vi "STAGE+mono+counter_edit1.vi"() -> ()   [LabVIEW 2017]
panel:
  in  "Integrating time, 10^-7 sec":dbl=10000000.0
  out "Timeout 2":bool
  in  "scan from":i32=2600
  in  "scan to":i32=4000
  in  "?":bool
  in  "Exit Labview":bool
  in  "step size":dbl=10.0 min=0.0
  in  "Name of measurement (optional)":string
  in  "?":bool
  out "Spectrum":waveform(dbl)(graph)
  out "Counts":i32
  in  "Background scan":bool=TRUE
  in  "value (0)":dbl=-9.0
  in  "number of disc steps":i32=1
  in  "Background scan 2":bool=TRUE
  out "Current WL Wavelength  2":u16 caption="Current Wavelength"
  out "Grt# 2":u8=1 min=1 max=3 step=1
  out "Blaze (nm)":u32=300
  out "Groove/mm":u32=1200
  in  "?":bool
  in  "Channel B Input":u16(ring)=2 items=["Input 1"=1, "Input 2"=2]
  in  "Trigger mode":u16(ring) items=["10 MHz"=0, "Input 2"=2, "Input T"=3]
  out "Current WL Wavelength":u16 caption="Current Wavelength"
  in  "Integrating time, 10^-7 sec":dbl=10000000.0
  in  "gate A mode (CW:0)":i16(slide) scale=0.0..2.0 scale format="%.2f"
  in  "Channel A Input":u16(ring)=1 items=["10 MHz", "Input 1"]
  in  "Time between measurements\n at one point (s)/Dwell Time":dbl=0.002 min=0.002 max=60.0 step=0.001
  in  "Number of Measurements\n to take at one point/ Number of Periods":u16=1 min=1 max=2000 step=1
  in  "Count Mode":u16(ring) items=["A,B for Preset T", "A-B for Preset T", "A+B for Preset T", "A for Preset B"]
  in  "GPIB address":string="23"
  out "Timeout":bool
  out "Serial":u32=12345
  out "Grt#":u8=1 min=1 max=3 step=1
  out "Blaze (nm)":u32=300
  out "Groove/mm":u32=1200
  out "time delay":u32=450000 min=1
  out "Mono port":T1(ring)
  in  "Get position":bool
  out "Position status":dbl format="%.3f"
  in  "Target position":dbl format="%.3f"
  in  "Move":bool
  in  "Motor OFF":bool
  in  "Motor ON":bool
  in  "Step Size [um]":i32=10
  in  "Axis":i32=1
  in  "Rep Rate [Hz]":dbl=500.0
  out "Shots":dbl
  in  "Averaging Time [s]":dbl=0.1
  out "Current Point":i32
  out "Slide":i32(slide) scale=0.0..100.0
  out "Current Position [mm]":dbl
  in  "Axis initial position [mm]":dbl
  out "Axis final Position [mm]":dbl
  in  "Data Points (100 default)":i32=100
  in  "Collect Data!":bool
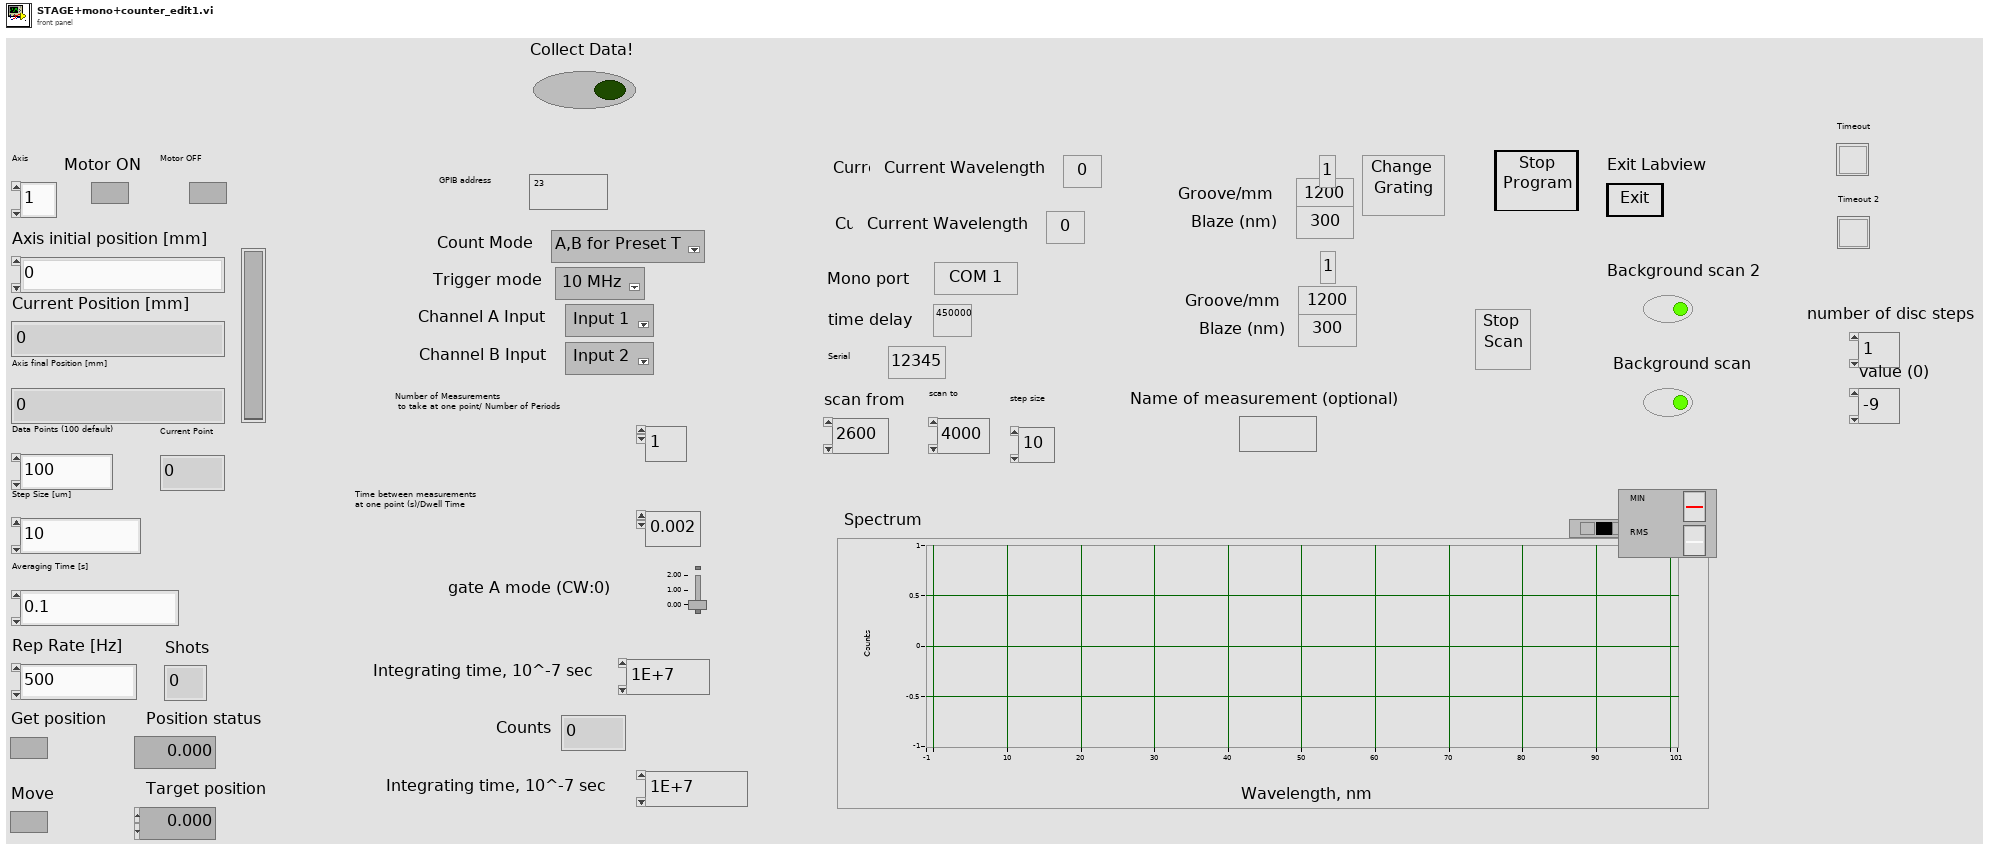
[diagram p1: front panel]
types:
  T1 = enum8{"COM 1", "COM 2", "COM 3", "COM 4", "COM 5", "COM 6", "COM 7", "COM 8", "COM 9"}
  T2 = cluster{"input XON/XOFF":bool, "input HW Handshake":bool, "input alt HW HShk":bool, "output XON/XOFF":bool, "output HW Handshake":bool, "output alt HW HShk":bool, "XOFF byte":u8, "XON byte":u8, "parity error byte":u16}
  T3 = enum16{"no parity", "odd parity", "even parity", "mark parity", "space parity"}
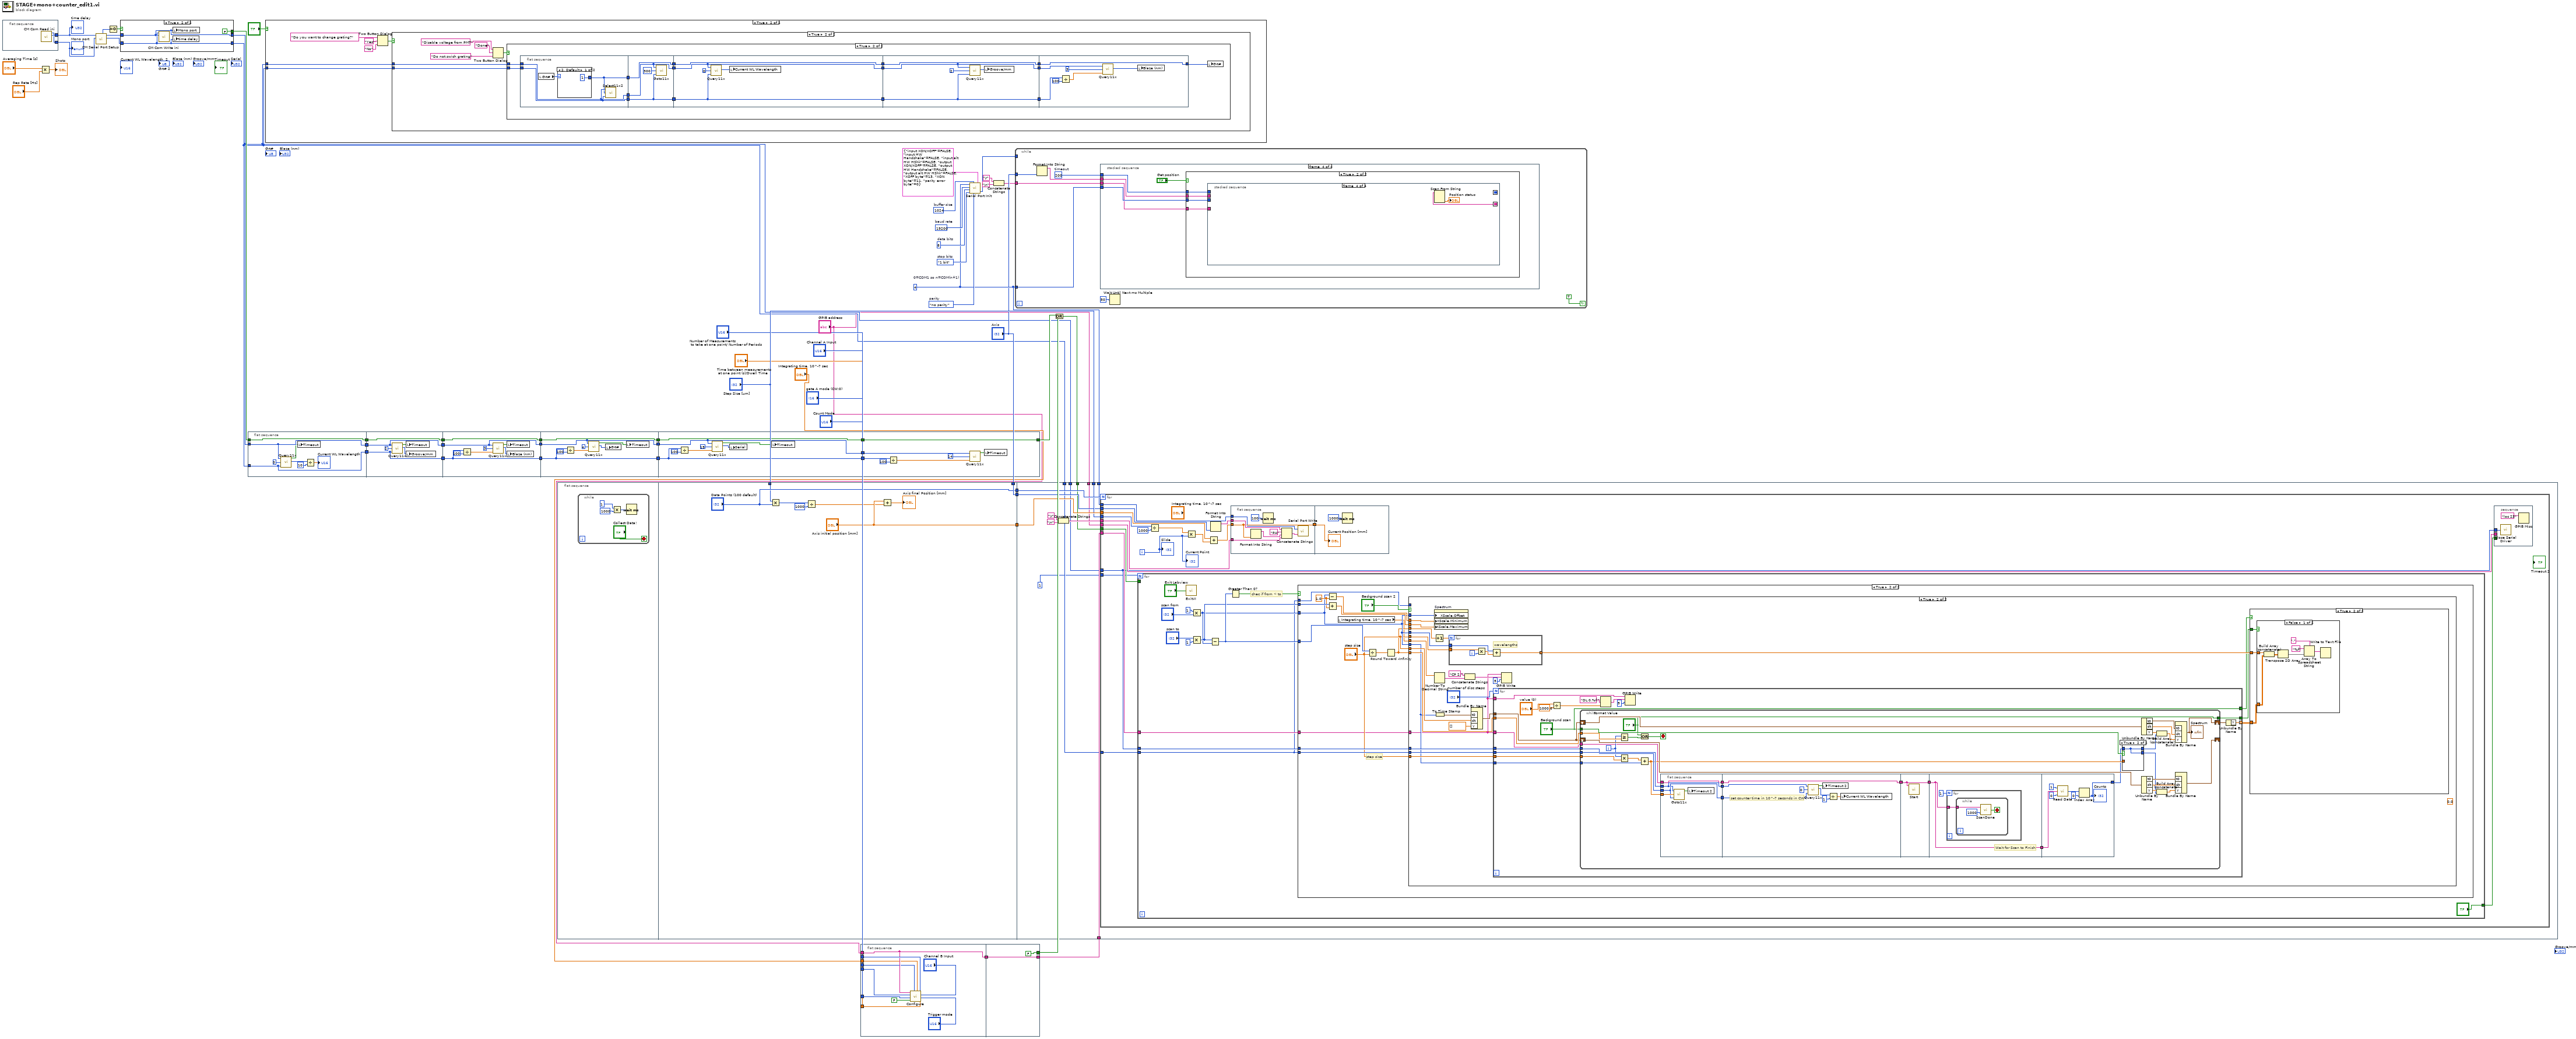
[diagram p0: block diagram]
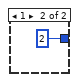
[diagram p5: hidden frame]
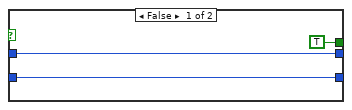
[diagram p6: hidden frame]
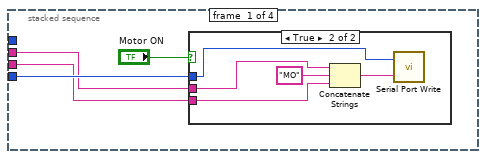
[diagram p7: hidden frame]
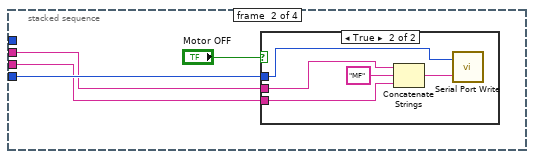
[diagram p9: hidden frame]
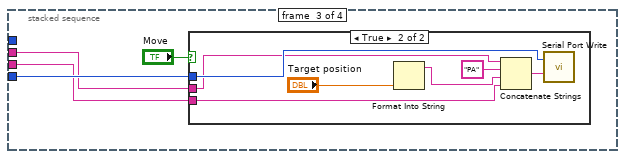
[diagram p11: hidden frame]
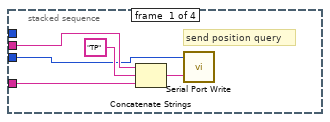
[diagram p14: hidden frame]
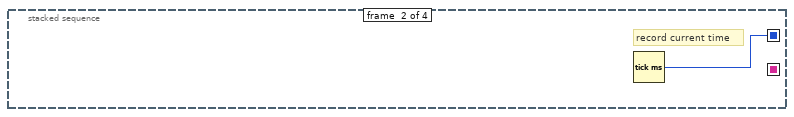
[diagram p15: hidden frame]
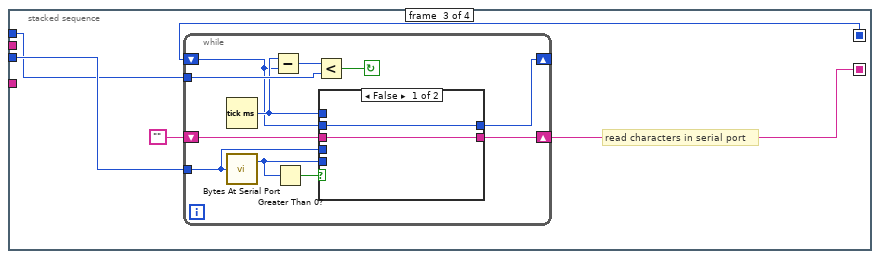
[diagram p16: hidden frame]
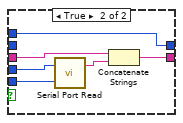
[diagram p17: hidden frame]
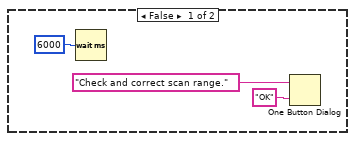
[diagram p18: hidden frame]
diagram:
  w46 = u32 19200  # baud rate
  w45 = u16 8  # data bits
  w44 = enum16{"1 bit", "1.5 bits", "2 bits"}."1 bit"  # stop bits
  w49 = T3."no parity"  # parity
  w43 = 4  # 0=COM1 so n=COM(n+1)
  w48 = u16 1024  # buffer size
  n1 = flat-sequence {
    tunnel: [w58] -> w21
    tunnel: [w57] -> w20
    frame #0 {
      n2 = call "CM Com Read ini.vi"() -> ("Mono port"=w57:T1, "time delay1"=w58:u32)  [unwired: 7 in]
    }
  }
  n3 = Multiply(x="Averaging Time [s]", y="Rep Rate [Hz]") -> (x*y=→"Shots":dbl)
  n4 = call "CM Serial Port Setup.vi"("COM port"=w20, "time delay"=w21) -> ("time delay1"=w16:u32, "DK port Out"=w17:T1, "error code"=w19:i32)  [unwired: 7 in]
  n5 = Equal To 0?(x=w19) -> (x = 0?=w18:bool)
  n6 = case shown="True" w18 {
    tunnel: w17 -> [w61 w64]
    tunnel: w16 -> [w60 w63]
    tunnel: [w61 w64] -> w3
    tunnel: [w60 w63] -> w2
    tunnel: [TRUE FALSE] -> w15
    frame False {
    }
    frame True {
      n7 = call "CM Com Write ini.vi"("time delay1"=w64, "Mono port"=w63) -> ()  [unwired: 7 in]
      n8 = local write "Mono port"(w64) -> ()
      n9 = local write "time delay"(w63) -> ()
    }
  }
  n10 = flat-sequence {
    tunnel: w2 -> [w70]
    tunnel: [w70] -> w37
    tunnel: w3 -> [w72]
    tunnel: [w72] -> w36
    tunnel: w15 -> [w68]
    tunnel: [w68] -> w35
    tunnel: w37 -> [w75]
    tunnel: [w75] -> w34
    tunnel: w36 -> [w77]
    tunnel: [w77] -> w33
    tunnel: w35 -> [w73]
    tunnel: [w73] -> w32
    tunnel: w34 -> [w85]
    tunnel: [w85] -> w31
    tunnel: w33 -> [w82]
    tunnel: [w82] -> w30
    tunnel: w32 -> [w79]
    tunnel: [w79] -> w29
    tunnel: w31 -> [w93]
    tunnel: [w93] -> w28
    tunnel: w30 -> [w90]
    tunnel: [w90] -> w27
    tunnel: w29 -> [w87]
    tunnel: [w87] -> w26
    tunnel: w28 -> [w101]
    tunnel: [w101] -> w25
    tunnel: w27 -> [w98]
    tunnel: [w98] -> w24
    tunnel: w26 -> [w95]
    tunnel: [w95] -> w23
    tunnel: w25 -> [w108]
    tunnel: w24 -> [w105]
    tunnel: [w103] -> w9
    tunnel: w23 -> [w103]
    frame #0 {
      n11 = call "Query11x.vi"("port number"=w72, "QUERY"=u16 0, "time delay"=w70) -> ("timeout"=w69:bool, "STATUS MESSAGE"=w67:u16)  [unwired: 2 out]
      n12 = local write "Timeout"(w69) -> ()
      n13 = Divide(x=w67, y=10 ("Numeric")) -> (x/y=→"Current WL Wavelength":dbl)
    }
    frame #1 {
      n14 = call "Query11x.vi"("port number"=w77, "QUERY"=u16 2, "time delay"=w75) -> ("timeout"=w74:bool, "STATUS MESSAGE"=w76:u16)  [unwired: 2 out]
      n15 = local write "Timeout"(w74) -> ()
      n16 = local write "Groove/mm"(w76) -> ()
    }
    frame #2 {
      n17 = Divide(x=w85, y=i16 100 ("device (1)")) -> (x/y=w83:dbl)
      n18 = call "Query11x.vi"("port number"=w82, "QUERY"=u16 3, "time delay"=w83) -> ("timeout"=w80:bool, "STATUS MESSAGE"=w81:u16)  [unwired: 2 out]
      n19 = local write "Timeout"(w80) -> ()
      n20 = local write "Blaze (nm)"(w81) -> ()
    }
    frame #3 {
      n21 = Divide(x=w93, y=i16 100 ("device (1)")) -> (x/y=w91:dbl)
      n22 = call "Query11x.vi"("port number"=w90, "QUERY"=u16 4, "time delay"=w91) -> ("timeout"=w88:bool, "STATUS MESSAGE"=w89:u16)  [unwired: 2 out]
      n23 = local write "Grt#"(w89) -> ()
      n24 = local write "Timeout"(w88) -> ()
    }
    frame #4 {
      n25 = Divide(x=w101, y=i16 100 ("device (1)")) -> (x/y=w99:dbl)
      n26 = call "Query11x.vi"("port number"=w98, "QUERY"=u16 19, "time delay"=w99) -> ("timeout"=w96:bool, "STATUS MESSAGE"=w97:u16)  [unwired: 2 out]
      n27 = local write "Serial"(w97) -> ()
      n28 = local write "Timeout"(w96) -> ()
    }
    frame #5 {
      n29 = Divide(x=w108, y=i16 100 ("device (1)")) -> (x/y=w106:dbl)
      n30 = call "Query11x.vi"("port number"=w105, "QUERY"=u16 14, "time delay"=w106) -> ("timeout"=w104:bool)  [unwired: 3 out]
      n31 = local write "Timeout"(w104) -> ()
    }
  }
  n32 = case shown="True" "?" {
    tunnel: w2 -> [_ w111]
    tunnel: w3 -> [_ w110]
    frame False {
    }
    frame True {
      n33 = Two Button Dialog(message="Do you want to change grating?", 1:"No" ("F button name (\"Cancel\")"), 2:"Yes" ("T button name (\"OK\")")) -> (T button?=w112:bool)
      n34 = case shown="True" w112 {
        tunnel: w111 -> [_ w117]
        tunnel: w110 -> [_ w116]
        frame False {
        }
        frame True {
          n35 = Two Button Dialog(message="Disable voltage from PMT", 1:"Do not swich grating" ("F button name (\"Cancel\")"), 2:"Done" ("T button name (\"OK\")")) -> (T button?=w118:bool)
          n36 = case shown="True" w118 {
            tunnel: w117 -> [_ w136]
            tunnel: w116 -> [_ w135]
            frame False {
            }
            frame True {
              n37 = flat-sequence {
                tunnel: w136 -> [w140]
                tunnel: [w140] -> w133
                tunnel: w135 -> [w139]
                tunnel: [w139] -> w132
                tunnel: [w137] -> w131
                tunnel: w133 -> [w144]
                tunnel: [w144] -> w130
                tunnel: w132 -> [w145]
                tunnel: [w145] -> w129
                tunnel: w131 -> [w143]
                tunnel: [w143] -> w128
                tunnel: w130 -> [w151]
                tunnel: [w151] -> w127
                tunnel: w129 -> [w150]
                tunnel: [w150] -> w126
                tunnel: w128 -> [w147]
                tunnel: [w147] -> w125
                tunnel: w127 -> [w154]
                tunnel: [w154] -> w124
                tunnel: w126 -> [w155]
                tunnel: [w155] -> w123
                tunnel: w125 -> [w152]
                tunnel: [w152] -> w122
                tunnel: w124 -> [w159]
                tunnel: w123 -> [w160]
                tunnel: [w157] -> w134
                tunnel: w122 -> [w157]
                frame #0 {
                  n38 = local read "Grt#"() -> (w138:u8)
                  n39 = case shown="2, Default" w138 {
                    tunnel: [1 2] -> w137
                    frame 2, Default {
                    }
                    frame 1 {
                    }
                  }
                  n40 = call "Select11x2.vi"("time delay"=w140, "NEW GRT?"=w137, "port number"=w139) -> ()  [unwired: 3 out]
                }
                frame #1 {
                  n41 = call "Goto11x.vi"("time delay"=w144, "WAVELENGTH"=u16 300, "port number"=w145) -> ()  [unwired: 3 out]
                }
                frame #2 {
                  n42 = call "Query11x.vi"("port number"=w150, "QUERY"=u16 0, "time delay"=w151) -> ("STATUS MESSAGE"=w148:u16)  [unwired: 3 out]
                  n43 = local write "Current WL Wavelength"(w148) -> ()
                }
                frame #3 {
                  n44 = call "Query11x.vi"("port number"=w155, "QUERY"=u16 2, "time delay"=w154) -> ("STATUS MESSAGE"=w153:u16)  [unwired: 3 out]
                  n45 = local write "Groove/mm"(w153) -> ()
                }
                frame #4 {
                  n46 = Divide(x=w159, y=i16 100 ("device (1)")) -> (x/y=w161:dbl)
                  n47 = call "Query11x.vi"("port number"=w160, "QUERY"=u16 3, "time delay"=w161) -> ("STATUS MESSAGE"=w158:u16)  [unwired: 3 out]
                  n48 = local write "Blaze (nm)"(w158) -> ()
                }
              }
              n49 = local write "Grt#"(w134) -> ()
            }
          }
        }
      }
    }
  }
  n50 = flat-sequence {
    tunnel: ["Data Points (100 default)"] -> w56
    tunnel: "Axis" -> [w175]
    tunnel: ["Axis initial position [mm]"] -> w55
    tunnel: "Step Size [um]" -> [w168]
    tunnel: [w175] -> w54
    tunnel: w56 -> [w189]
    tunnel: w55 -> [w188]
    tunnel: "Step Size [um]" -> [w187]
    tunnel: w54 -> [w186]
    tunnel: w43 -> [w182]
    tunnel: w5 -> [w181]
    tunnel: w4 -> [w180]
    tunnel: w3 -> [w179]
    tunnel: w2 -> [w178]
    tunnel: "GPIB address" -> [w177]
    frame #0 {
      n51 = while {
        stop <- "Collect Data!" stop-if-true
        n52 = Multiply(x=1, y=1000) -> (x*y=w167:i32)
        n53 = Wait (ms)(milliseconds to wait=w167) -> ()  [unwired: 1 out]
      }
    }
    frame #1 {
      n54 = Multiply(x=w168, y="Data Points (100 default)") -> (x*y=w171:i32)
      n55 = Divide(x=w171, y=1000) -> (x/y=w170:dbl)
      n56 = Add(x="Axis initial position [mm]", y=w170) -> (x+y=→"Axis final Position [mm]":dbl)
    }
    frame #2 {
      n57 = Concatenate Strings("\r", "\n") -> (w183:string)
      n58 = for {
        N: w189 -> [_]
        tunnel: w188 -> [w207]
        tunnel: w187 -> [w203]
        tunnel: w186 -> [w200]
        tunnel: w183 -> [w197]
        tunnel: w182 -> [w198]
        tunnel: w181 -> [w195]
        tunnel: w180 -> [w194]
        tunnel: w179 -> [w191]
        tunnel: w178 -> [w193]
        tunnel: w177 -> [w192]
        tunnel: 1 -> [w190]
        i -> [w208]
        n59 = for {
          N: w190 -> [_]
          tunnel: w191 -> [w218]
          tunnel: w193 -> [w209]
          tunnel: ["?"] -> w196
          tunnel: w194 -> [_]
          tunnel: w195 -> [w216]
          # "chec if from < to"
          n60 = call "ExitVI.vi"("Exit Labview"="Exit Labview") -> ()
          n61 = Multiply(x=1, y="scan from") -> (x*y=w211:i32)
          n62 = Multiply(x="scan to", y=1) -> (x*y=w213:i32)
          n63 = Subtract(x=w213, y=w211) -> (x-y=w221:i32)
          n64 = Greater Than 0?(x=w221) -> (x > 0?=w217:bool)
          n65 = case shown="True" w217 {
            tunnel: w221 -> [_ w239]
            tunnel: w218 -> [_ w237]
            tunnel: w209 -> [_ w236]
            tunnel: w213 -> [_ w235]
            tunnel: w211 -> [_ w231]
            tunnel: w216 -> [_ w228]
            tunnel: w209 -> [_ w225]
            frame False {
              n66 = Wait (ms)(milliseconds to wait=u32 6000) -> ()  [unwired: 1 out]
              n67 = One Button Dialog(message="Check and correct scan range.", button name ("OK")="OK") -> ()  [unwired: 1 out]
            }
            frame True {
              w233 = 1.0 ("x")
              # "step size"
              n68 = Subtract(x=w231, y=w233) -> (x-y=w232:dbl)
              n69 = Add(x=w235, y=w233) -> (x+y=w234:dbl)
              n70 = local read "Integrating time, 10^-7 sec"() -> (w227:dbl)
              n71 = Divide(x=w239, y="step size") -> (x/y=w238:dbl)
              n72 = Round Toward -Infinity(1:w238) -> (0:w229:dbl)
              n73 = case shown="True" "Background scan 2" {
                tunnel: w231 -> [_ w249]
                tunnel: "step size" -> [_ w266]
                tunnel: w229 -> [_ w263]
                tunnel: w237 -> [_ w265]
                tunnel: w236 -> [_ w264]
                tunnel: w227 -> [_ w243]
                tunnel: "step size" -> [_ w260]
                tunnel: w234 -> [_ w258]
                tunnel: w232 -> [_ w259]
                tunnel: w231 -> [_ w248]
                tunnel: w231 -> [_ w255]
                tunnel: "step size" -> [_ w256]
                tunnel: w229 -> [_ w254]
                tunnel: w228 -> [_ w240]
                tunnel: w225 -> [_ _]
                frame False {
                }
                frame True {
                  (unwired) 0.0 ("element")
                  n74 = Increment(x=w254) -> (x+1=w253:dbl)
                  n75 = property on="Spectrum" class="WFGraph (strict)"("XScale.Offset"=w248, "XScale.Minimum"=w259, "XScale.Maximum"=w258) -> ()  [unwired: 2 in, 2 out]
                  n76 = Number To Decimal String(number=w243) -> (decimal integer string=w246:string)  [unwired: 1 in]
                  n77 = To Time Stamp(1:w249) -> (0:w261:timestamp)
                  n78 = for {
                    N: w253 -> [_]
                    tunnel: w256 -> [w394]
                    tunnel: w255 -> [w392]
                    tunnel: [w390] -> w252 mode=indexing
                    i -> [w393]
                    # "wavelengths"
                    n79 = Multiply(x=w394, y=w393) -> (x*y=w391:dbl)
                    n80 = Add(x=w392, y=w391) -> (x+y=w390:dbl)
                  }
                  n81 = Concatenate Strings("CP 2,", w246) -> (w244:string)
                  n82 = Bundle By Name("t0"=w261, "dt"=w260, "Y"=dbl[] []) -> (w257:waveform(dbl))  [unwired: 1 in]
                  n83 = for {
                    N: "number of disc steps" -> [_]
                    tunnel: w266 -> [w284]
                    tunnel: w265 -> [w283]
                    tunnel: w264 -> [w282]
                    tunnel: w263 -> [w281]
                    tunnel: w257 -> [w280]
                    tunnel: [w279] -> w251
                    tunnel: ["Background scan"] -> w250
                    tunnel: w249 -> [w277]
                    tunnel: w240 -> [w276]
                    tunnel: [w274] -> w241 mode=indexing
                    tunnel: w240 -> [w270]
                    n84 = Divide(x="value (0)", y=1000.0) -> (x/y=w267:dbl)
                    n85 = while {
                      tunnel: w277 -> [w301]
                      tunnel: w284 -> [w318]
                      tunnel: w283 -> [w316]
                      tunnel: w282 -> [w315]
                      tunnel: w281 -> [w314]
                      shift-right: [w293] -> w275
                      shift-left: w280 -> [w312]
                      shift-right: [w294] -> _
                      shift-left: w280 -> [w307]
                      tunnel: ["?"] -> w279
                      tunnel: "Background scan" -> [w300]
                      tunnel: w276 -> [w292]
                      i -> [w306]
                      stop <- w313 stop-if-true
                      n86 = Greater Or Equal?(x=w306, y=w314) -> (x >= y?=w295:bool)
                      n87 = Multiply(x=w306, y=w318) -> (x*y=w317:dbl)
                      n88 = Or(x="?", y=w295) -> (x .or. y?=w313:bool)
                      n89 = Add(x=w317, y=w301) -> (x+y=w297:dbl)
                      n90 = flat-sequence {
                        tunnel: w297 -> [w323]
                        tunnel: w316 -> [w322]
                        tunnel: [w322] -> w290
                        tunnel: w315 -> [w321]
                        tunnel: [w321] -> w289
                        tunnel: w292 -> [w319]
                        tunnel: [w319] -> w288
                        tunnel: w290 -> [w330]
                        tunnel: w289 -> [w329]
                        tunnel: w288 -> [w327]
                        tunnel: [w327] -> w287
                        tunnel: w287 -> [w332]
                        tunnel: [w332] -> w286
                        tunnel: w286 -> [w333]
                        tunnel: [w333] -> w285
                        tunnel: w285 -> [w340]
                        tunnel: [w339] -> w291
                        frame #0 {
                          n91 = call "Goto11x.vi"("time delay"=w321, "WAVELENGTH"=w323, "port number"=w322) -> ("timeout"=w320:bool)  [unwired: 2 out]
                          n92 = local write "Timeout 2"(w320) -> ()
                        }
                        frame #1 {
                          # "set counter time in 10^-7 seconds in CW"
                          n93 = call "Query11x.vi"("port number"=w330, "QUERY"=0, "time delay"=w329) -> ("timeout"=w328:bool, "STATUS MESSAGE"=w326:u16)  [unwired: 2 out]
                          n94 = local write "Timeout 2"(w328) -> ()
                          n95 = Divide(x=w326, y=1) -> (x/y=w325:dbl)
                          n96 = local write "Current WL Wavelength"(w325) -> ()
                        }
                        frame #2 {
                          n97 = call "Start.vi"("GPIB Address"=w332) -> ()  [unwired: 9 in]
                        }
                        frame #3 {
                          # "Wait for Scan to Finish"
                          n98 = for {
                            N: 1 -> [_]
                            tunnel: w333 -> [w335]
                            n99 = while {
                              tunnel: w335 -> [w336]
                              stop <- w338 stop-if-true
                              n100 = call "ScanDone.vi"("Wait (ms)"=1000, "GPIB Address"=w336) -> ("Scan Finished?"=w338:bool)
                            }
                          }
                        }
                        frame #4 {
                          n101 = call "Read Data.vi"("Channel Number"=0, "GPIB Address"=w340, "Number of Datapoints"=1) -> ("Data"=w341:i32[])
                          n102 = Index Array(array=w341, index=0) -> (element=w339:i32)
                          "Counts" <- w339
                        }
                      }
                      n103 = case shown="True" w300 {
                        tunnel: [w345 w346] -> w299
                        tunnel: [w345 w346] -> w298
                        tunnel: w297 -> [_ _]
                        tunnel: w291 -> [w345 w346]
                        frame False {
                        }
                        frame True {
                        }
                      }
                      n104 = Unbundle By Name(w312) -> ("t0"=w310:timestamp, "dt"=w311:dbl, "Y"=w305:dbl[])
                      n105 = Unbundle By Name(w307) -> ("t0"=w308:timestamp, "dt"=w309:dbl, "Y"=w303:dbl[])
                      n106 = Build Array (concatenate)(w305, w299) -> (w304:dbl[])
                      n107 = Build Array (concatenate)(w303, w298) -> (w302:dbl[])
                      n108 = Bundle By Name("t0"=w310, "dt"=w311, "Y"=w304) -> (w293:waveform(dbl))  [unwired: 1 in]
                      "Spectrum" <- w293
                      n109 = Bundle By Name("t0"=w308, "dt"=w309, "Y"=w302) -> (w294:waveform(dbl))  [unwired: 1 in]
                    }
                    n110 = Format Value(format string="DL 0,%f;", value (0)=w267) -> (output string=w272:string)  [unwired: 1 in]
                    n111 = GPIB Write(0:w270, 1:w272, 2:i16 5 ("mode (0)")) -> ()  [unwired: 2 in, 2 out]
                    n112 = Unbundle By Name(w275) -> ("Y"=w274:dbl[])
                  }
                  n113 = GPIB Write(0:w240, 1:w244, 2:i16 5 ("mode (0)")) -> ()  [unwired: 2 in, 2 out]
                  n114 = case shown="True" w250 {
                    tunnel: w252 -> [w349 w381]
                    tunnel: w251 -> [w348 w382]
                    tunnel: w241 -> [w347 w380]
                    frame False {
                      n115 = case shown="False" w348 {
                        tunnel: w349 -> [w354 _]
                        tunnel: w347 -> [w350 _]
                        frame False {
                          w356 = "\r\n"
                          n116 = Build Array (concatenate)(w354, w350) -> (w353:dbl[][])
                          n117 = Transpose 2D Array(2D array=w353) -> (transposed array=w352:dbl[][])
                          n118 = local read "Integrating time, 10^-7 sec"() -> (w351:dbl)
                          n119 = Array To Spreadsheet String(delimiter (Tab)=",", array=w352, 3:"%f" ("format string")) -> (spreadsheet string=w355:string)
                          n120 = local read "Blaze (nm)"() -> (w359:u32)
                          n121 = local read "Grt#"() -> (w360:u8)
                          n122 = Get Date/Time In Seconds() -> (seconds since 1Jan1904=w377:timestamp)
                          n123 = Format Date/Time String(time format string (%c)="%Y-%b-%d %H:%M:%S", seconds (now)=w377) -> (date/time string=w374:string)  [unwired: 1 in]
                          n124 = Number To Decimal String(number=w351) -> (decimal integer string=w370:string)  [unwired: 1 in]
                          n125 = Number To Decimal String(number=w360) -> (decimal integer string=w367:string)  [unwired: 1 in]
                          n126 = Number To Decimal String(number=w359) -> (decimal integer string=w364:string)  [unwired: 1 in]
                          n127 = call <vilib>:"Space Constant.vi"() -> ("String"=w363:string)
                          n128 = Concatenate Strings("Measurement: ", "Name of measurement (optional)", w356, "Data was taken on ", w374, w356, "Integration Time is ", w370, w363, "ms", w356, "Monochromator gratng # ", w367, "; ", "blazed for ", w364, w363, "nm", w356, "gain voltage is ", " volts", w356, w356, w355) -> (w361:string)
                          n129 = Write to Text File(text=w361) -> ()  [unwired: 3 in, 3 out]
                        }
                        frame True {
                        }
                      }
                    }
                    frame True {
                      n130 = case shown="False" w382 {
                        tunnel: w381 -> [w384 _]
                        tunnel: w380 -> [w383 _]
                        frame False {
                          n131 = Build Array (concatenate)(w384, w383) -> (w387:dbl[][])
                          n132 = Transpose 2D Array(2D array=w387) -> (transposed array=w386:dbl[][])
                          n133 = Array To Spreadsheet String(delimiter (Tab)=",", array=w386, 3:"%f" ("format string")) -> (spreadsheet string=w385:string)
                          n134 = Write to Text File(text=w385) -> ()  [unwired: 3 in, 3 out]
                        }
                        frame True {
                        }
                      }
                    }
                  }
                }
              }
            }
          }
        }
        n135 = Divide(x=w203, y=1000) -> (x/y=w202:dbl)
        n136 = Multiply(x=w202, y=w208) -> (x*y=w206:dbl)
        n137 = Add(x=w207, y=w206) -> (x+y=w205:dbl)
        n138 = Format Into String(w200) -> (resulting string=w199:string)  [unwired: 3 in, 1 out]
        n139 = flat-sequence {
          tunnel: w205 -> [w399]
          tunnel: [w399] -> w201
          tunnel: w197 -> [w401]
          tunnel: w199 -> [w400]
          tunnel: w198 -> [w397]
          tunnel: w201 -> [w405]
          frame #0 {
            n140 = Format Into String(w399) -> (resulting string=w398:string)  [unwired: 3 in, 1 out]
            n141 = Wait (ms)(milliseconds to wait=u32 100) -> ()  [unwired: 1 out]
            n142 = Concatenate Strings(w400, "PA" ("Substring"), w398, w401) -> (w403:string)
            n143 = call <vilib>:"Serial Port Write.vi"("string to write"=w403, "port number"=w397) -> ()  [unwired: 1 out]
          }
          frame #1 {
            n144 = Wait (ms)(milliseconds to wait=u32 1000) -> ()  [unwired: 1 out]
            "Current Position [mm]" <- w405
          }
        }
        n145 = stacked-sequence {
          tunnel: w196 -> [_]
          tunnel: w191 -> [w396]
          tunnel: w192 -> [_]
          frame #0 {
            n146 = call <vilib>:"Close Serial Driver.vi"("port number"=w396) -> ()  [unwired: 1 out]
            n147 = GPIB Misc(0:"loc 23" ("command string")) -> ()  [unwired: 1 in, 3 out]
          }
        }
        "Current Point" <- w208
        "Slide" <- w208
      }
    }
  }
  n148 = flat-sequence {
    tunnel: "GPIB address" -> [w414]
    tunnel: [w414] -> w22
    tunnel: "Count Mode" -> [w415]
    tunnel: "Number of Measurements\n to take at one point/ Number of Periods" -> [w412]
    tunnel: "Time between measurements\n at one point (s)/Dwell Time" -> [w411]
    tunnel: "Channel A Input" -> [w416]
    tunnel: "gate A mode (CW:0)" -> [w408]
    tunnel: "Integrating time, 10^-7 sec" -> [w407]
    tunnel: w22 -> [w417]
    tunnel: [w417] -> w5
    tunnel: [FALSE] -> w10
    frame #0 {
      n149 = call "Configure.vi"("Dwell Time (s)"=w411, "Channel T Input"="Trigger mode", "Channel B Input"="Channel B Input", "Channel A Input"=w416, "Integrating time, 10^-7 sec"=w407, "gate mode (CW:0)"=w408, "Scan End Mode"=FALSE, "Number of Periods"=w412, "Count Mode"=w415, "GPIB Address"=w414) -> ()
    }
    frame #1 {
    }
  }
  n150 = call <vilib>:"Serial Port Init.vi"("flow control etc."=T2 {"input XON/XOFF"=FALSE, "input HW Handshake"=FALSE, "input alt HW HShk"=FALSE, "output XON/XOFF"=FALSE, "output HW Handshake"=FALSE, "output alt HW HShk"=FALSE, "XOFF byte"=13, "XON byte"=11, "parity error byte"=0}, "parity"=w49, "buffer size"=w48, "stop bits"=w44, "data bits"=w45, "baud rate"=w46, "port number"=w43) -> ("error code"=w42:i32)
  n151 = Concatenate Strings("\r", "\n") -> (w38:string)
  n152 = while {
    tunnel: w43 -> [w421]
    tunnel: w38 -> [w422]
    tunnel: w42 -> [_]
    tunnel: "Axis" -> [w419]
    stop <- TRUE continue-if-true
    w420 = u32 200  # timeout
    n153 = Format Into String(w419) -> (resulting string=w423:string)  [unwired: 3 in, 1 out]
    n154 = stacked-sequence {
      tunnel: w423 -> [w427 w437 w446 w458]
      tunnel: w422 -> [w426 w436 w445 w455]
      tunnel: w421 -> [w428 w438 w447 w457]
      tunnel: w420 -> [_ _ _ w456]
      frame #0 {
        n155 = case shown="True" "Motor ON" {
          tunnel: w428 -> [_ w434]
          tunnel: w427 -> [_ w431]
          tunnel: w426 -> [_ w430]
          frame False {
          }
          frame True {
            n156 = Concatenate Strings(w431, "MO" ("Substring"), w430) -> (w432:string)
            n157 = call <vilib>:"Serial Port Write.vi"("string to write"=w432, "port number"=w434) -> ()  [unwired: 1 out]
          }
        }
      }
      frame #1 {
        n158 = case shown="True" "Motor OFF" {
          tunnel: w438 -> [_ w443]
          tunnel: w437 -> [_ w440]
          tunnel: w436 -> [_ w439]
          frame False {
          }
          frame True {
            n159 = Concatenate Strings(w440, "MF" ("Substring"), w439) -> (w441:string)
            n160 = call <vilib>:"Serial Port Write.vi"("string to write"=w441, "port number"=w443) -> ()  [unwired: 1 out]
          }
        }
      }
      frame #2 {
        n161 = case shown="True" "Move" {
          tunnel: w447 -> [_ w454]
          tunnel: w446 -> [_ w451]
          tunnel: w445 -> [_ w450]
          frame False {
          }
          frame True {
            n162 = Format Into String("Target position") -> (resulting string=w448:string)  [unwired: 3 in, 1 out]
            n163 = Concatenate Strings(w451, "PA" ("Substring"), w448, w450) -> (w452:string)
            n164 = call <vilib>:"Serial Port Write.vi"("string to write"=w452, "port number"=w454) -> ()  [unwired: 1 out]
          }
        }
      }
      frame #3 {
        n165 = case shown="True" "Get position" {
          tunnel: w458 -> [_ w463]
          tunnel: w457 -> [_ w462]
          tunnel: w456 -> [_ w461]
          tunnel: w455 -> [_ w460]
          frame False {
          }
          frame True {
            n166 = stacked-sequence {
              seq-local: [_ w469 _ _] -> [_ _ w471 _]
              seq-local: [_ _ w470 _] -> [_ _ _ w495]
              tunnel: w463 -> [w466 _ _ _]
              tunnel: w462 -> [w465 _ w474 _]
              tunnel: w461 -> [_ _ w472 _]
              tunnel: w460 -> [w464 _ _ _]
              frame #0 {
                # "send position query"
                n167 = Concatenate Strings(w466, "TP" ("Substring"), w464) -> (w467:string)
                n168 = call <vilib>:"Serial Port Write.vi"("string to write"=w467, "port number"=w465) -> ()  [unwired: 1 out]
              }
              frame #1 {
                # "record current time"
                n169 = Tick Count (ms)() -> (millisecond timer value=w469:u32)
              }
              frame #2 {
                # "read characters in serial port"
                n170 = while {
                  shift-left: w471 -> [w475]
                  shift-right: [w476] -> _
                  tunnel: w472 -> [w479]
                  shift-left: "" -> [w482]
                  shift-right: [w481] -> w470
                  tunnel: w474 -> [w483]
                  stop <- w478 continue-if-true
                  n171 = Tick Count (ms)() -> (millisecond timer value=w477:u32)
                  n172 = call <vilib>:"Bytes At Serial Port.vi"("port number"=w483) -> ("byte count"=w484:u32)  [unwired: 1 out]
                  n173 = Subtract(x=w477, y=w475) -> (x-y=w480:u32)
                  n174 = Greater Than 0?(x=w484) -> (x > 0?=w485:bool)
                  n175 = Less?(x=w480, y=w479) -> (x < y?=w478:bool)
                  n176 = case shown="False" w485 {
                    tunnel: w484 -> [_ w493]
                    tunnel: w483 -> [_ w492]
                    tunnel: w482 -> [w487 w490]
                    tunnel: [w487 w489] -> w481
                    tunnel: [w486 w488] -> w476
                    tunnel: w477 -> [_ w488]
                    tunnel: w475 -> [w486 _]
                    frame False {
                    }
                    frame True {
                      n177 = call <vilib>:"Serial Port Read.vi"("requested byte count"=w493, "port number"=w492) -> ("string read"=w491:string)  [unwired: 1 out]
                      n178 = Concatenate Strings(w490, w491) -> (w489:string)
                    }
                  }
                }
              }
              frame #3 {
                n179 = Scan From String(input string=w495) -> (output 1=→"Position status":dbl)  [unwired: 4 in, 3 out]
              }
            }
          }
        }
      }
    }
    n180 = Wait Until Next ms Multiple(millisecond multiple=u32 50) -> ()  [unwired: 1 out]
  }
  n181 = Or(x=w9, y=w10) -> (x .or. y?=w4:bool)
  "Mono port" <- w20
  "time delay" <- w21
